vi "Example Arduino Serial.vi"() -> ()   [LabVIEW 2014]
panel:
  out "Error Out":errorcluster
  in  "Error In":errorcluster
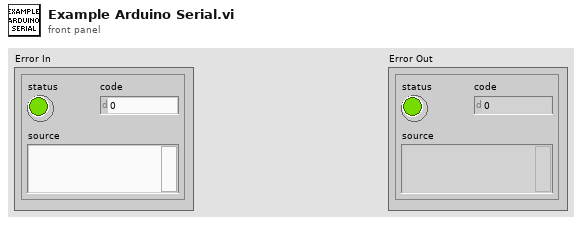
[diagram p1: front panel]
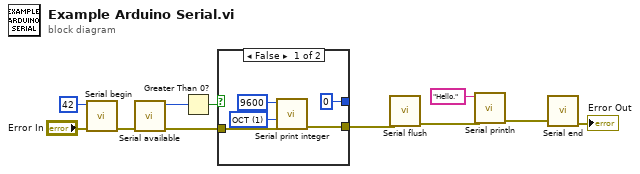
[diagram p0: block diagram]
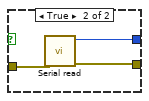
[diagram p2: hidden frame]
diagram:
  n1 = call "Serial begin.vi"("Error In"="Error In", "speed (Bd)"=42) -> ("Error Out"=w9:errorcluster)  [unwired: 9 in]
  n2 = call "Serial available.vi"("Error In"=w9) -> ("Error Out"=w6:errorcluster, "available bytes"=w8:i32)  [unwired: 9 in]
  n3 = Greater Than 0?(x=w8) -> (x > 0?=w7:bool)
  n4 = case shown="False" w7 {
    tunnel: w6 -> [w16 w19]
    tunnel: [0 ("data") w18] -> _
    tunnel: [w13 w17] -> w5
    frame False {
      w12 = u16 1 items=["BIN", "OCT", "HEX", "DEC"] ("format")
      n5 = call "Serial print integer.vi"("Error In"=w16, "format"=w12, "number to print"=9600 ("speed (Bd)")) -> ("Error Out"=w13:errorcluster)  [unwired: 8 in]
    }
    frame True {
      n6 = call "Serial read.vi"("Error In"=w19) -> ("Error Out"=w17:errorcluster, "data"=w18:i32)  [unwired: 9 in]
    }
  }
  n7 = call "Serial flush.vi"("Error In"=w5) -> ("Error Out"=w4:errorcluster)  [unwired: 10 in]
  n8 = call "Serial println.vi"("Error In"=w4, "string in"="Hello.") -> ("Error Out"=w3:errorcluster)  [unwired: 9 in]
  n9 = call "Serial end.vi"("Error In"=w3) -> ("Error Out"=→"Error Out":errorcluster)  [unwired: 10 in]
